vi "Get All Package BuildSpecs.vi"(8 "error in (no error)":errorcluster, 11 "LabVIEW project filepath":path) -> (0 "error out":errorcluster, 1 "package build spec names":string[](array[string]), 2 "all package build spec refs":refnum<vi>[](array[refnum]), 3 "project ref out":refnum<vi>, 4 "# of package build specs":i32)   [LabVIEW 2018, in "NIPKG BuildSpec API.lvlib"]
uses:
  NIPKG BuildSpec API.lvlib
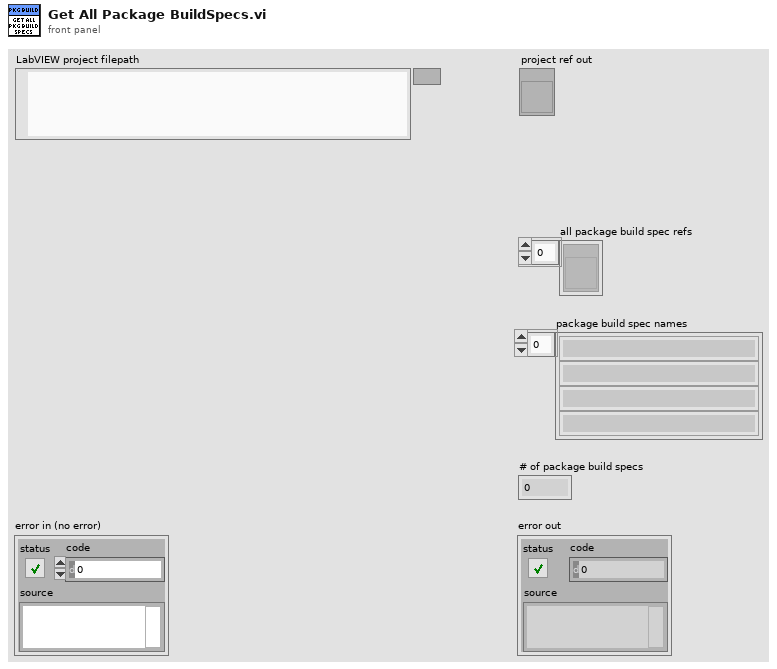
[diagram p1: front panel]
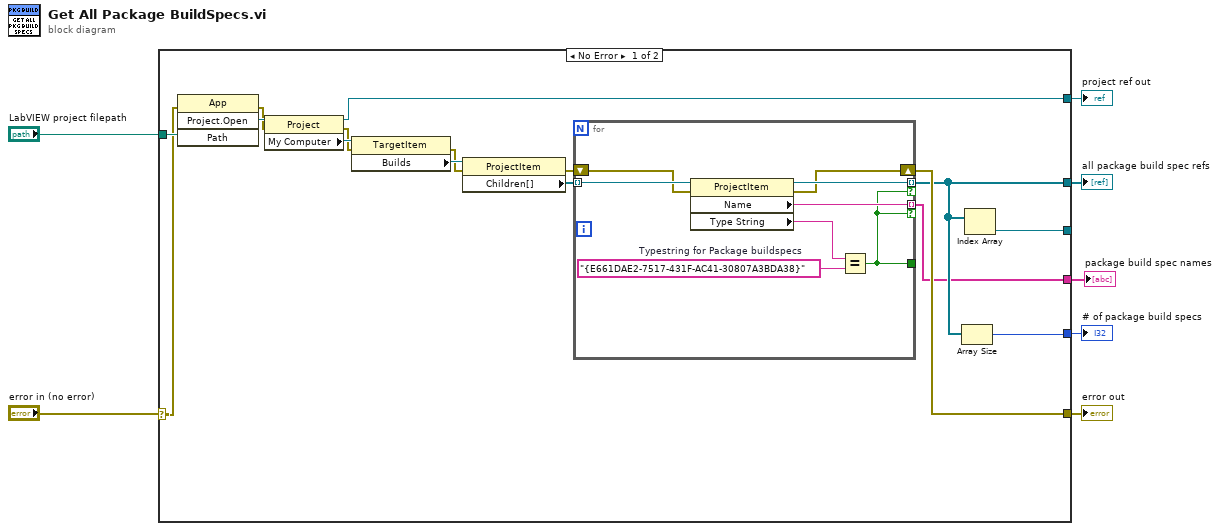
[diagram p0: block diagram]
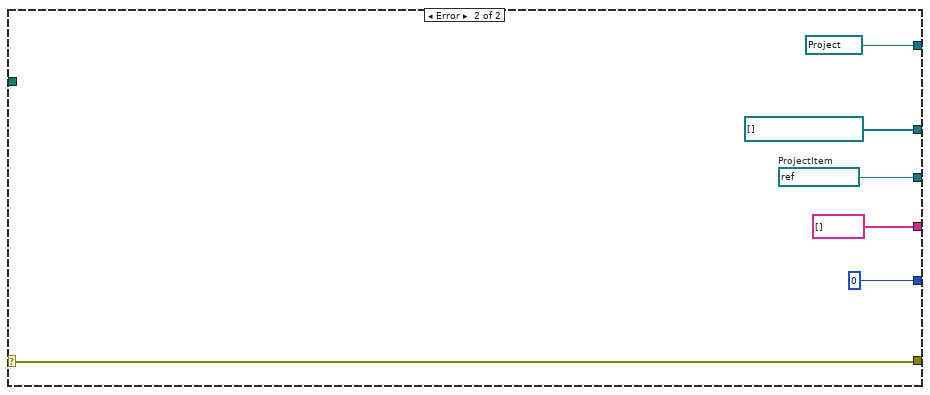
[diagram p2: hidden frame]
diagram:
  n1 = case shown="No Error" "error in (no error)" {
    selector: "error in (no error)" -> [w17 w37]
    tunnel: "LabVIEW project filepath" -> [w19 _]
    tunnel: [w10 refnum<vi>[] []] -> w6
    tunnel: [w18 0] -> w5
    tunnel: [w12 w37] -> w3
    tunnel: [w11 refnum<vi> refnum ("Project:Open")] -> w2
    tunnel: [w9 w33] -> _
    tunnel: [w8 string[] []] -> w1
    frame No Error {
      n2 = invoke class="App" method="Project.Open"(error in=w17, "Path"=w19) -> (error out=w16:errorcluster, "Project:Open"=w23:refnum<vi>)  [unwired: 2 in, 2 out]
      n3 = property class="Project"(reference=w23, error in=w16) -> (reference out=w11:refnum<vi>, error out=w15:errorcluster, "My Computer"=w22:refnum<vi>)
      n4 = property class="TargetItem"(reference=w22, error in=w15) -> (error out=w14:errorcluster, "Builds"=w21:refnum<vi>)  [unwired: 1 out]
      n5 = property class="ProjectItem"(reference=w21, error in=w14) -> (error out=w13:errorcluster, "Children[]"=w20:refnum<vi>[])  [unwired: 1 out]
      n6 = for {
        tunnel: w20 -> [w31] mode=indexing
        tunnel: [w30] -> w8 mode=indexing if=w24
        tunnel: [w27] -> w10 mode=indexing if=w24
        tunnel: [w24] -> _
        shift-right: [w25] -> w12
        shift-left: w13 -> [w26]
        w28 = "{E661DAE2-7517-431F-AC41-30807A3BDA38}"  # Typestring for Package buildspecs
        n7 = property class="ProjectItem"(reference=w31, error in=w26) -> (reference out=w27:refnum<vi>, error out=w25:errorcluster, "Name"=w30:string, "Type String"=w29:string)
        n8 = Equal?(x=w29, y=w28) -> (x = y?=w24:bool)
      }
      n9 = Array Size(array=w10) -> (size(s)=w18:i32)
      n10 = Index Array(array=w10) -> (element=w9:refnum<vi>)  [unwired: 1 in]
    }
    frame Error {
      w33 = refnum<vi> refnum  # ProjectItem
    }
  }
  "all package build spec refs" <- w6
  "# of package build specs" <- w5
  "error out" <- w3
  "project ref out" <- w2
  "package build spec names" <- w1
